vi "Manual Forearm Control.vi"() -> ()   [LabVIEW 2017]
panel:
  out "New Forearm\nAngle":dbl
  out "New Backarm\nAngle":dbl
  in  "Current Backarm\nAngle":dbl
  in  "Current Forearm\nAngle":dbl
  in  "Forearm Angle\nChange":dbl
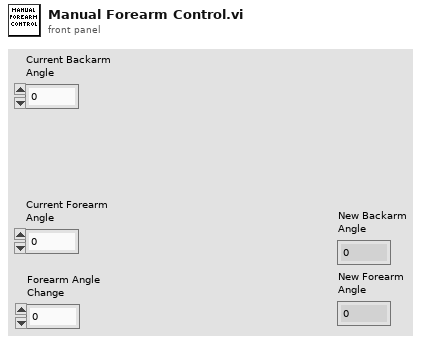
[diagram p1: front panel]
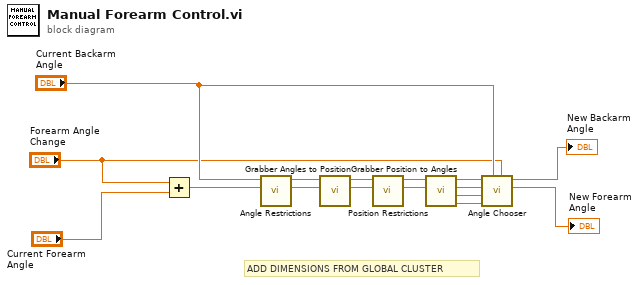
[diagram p0: block diagram]
diagram:
  # "ADD DIMENSIONS FROM GLOBAL CLUSTER"
  n1 = Add(x="Forearm Angle\nChange", y="Current Forearm\nAngle") -> (x+y=w4:dbl)
  n2 = call "Angle Restrictions.vi"("Forearm Angle 1"=w4, "Backarm Angle 1"="Current Backarm\nAngle") -> ("modified Forearm Angle 1"=w14:dbl, "modified Backarm Angle 1"=w15:dbl)  [unwired: 8 in]
  n3 = call "Grabber Angles to Position.vi"("Forearm Angle Degrees"=w14, "Backarm Angle Degrees"=w15) -> ("Y Final"=w12:dbl, "X Final"=w13:dbl)  [unwired: 8 in]
  n4 = call "Position Restrictions.vi"("newY"=w12, "newX"=w13) -> ("modified Y"=w10:dbl, "modified X"=w11:dbl)  [unwired: 8 in]
  n5 = call "Grabber Position to Angles.vi"("Y Initial"=w10, "X Initial"=w11) -> ("Forearm Angle\nDegrees 2"=w6:dbl, "Backarm Angle\nDegrees 2"=w7:dbl, "Forearm Angle\nDegrees 1"=w8:dbl, "Backarm Angle\nDegrees 1"=w9:dbl)  [unwired: 6 in]
  n6 = call "Angle Chooser.vi"("Forearm Angle Initial"="Forearm Angle\nChange", "Backarm Angle Initial"="Current Backarm\nAngle", "Forearm Angle 2"=w6, "Backarm Angle 2"=w7, "Forearm Angle 1"=w8, "Backarm Angle 1"=w9) -> ("final Forearm Angle"=→"New Forearm\nAngle":dbl, "final Backarm Angle"=→"New Backarm\nAngle":dbl)  [unwired: 4 in]
